vi "Example of fetch current git version code.vi"() -> ()   [LabVIEW 2016]
panel:
  out "Fetch error?":bool
  out "error out":errorcluster
  out "Version:":string
  # "Run the VI to get version code from the most recent tag with\ngit describe command in this containing folder"
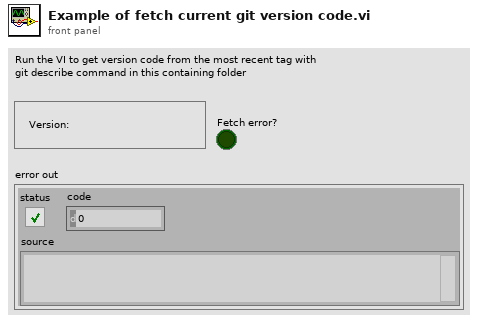
[diagram p1: front panel]
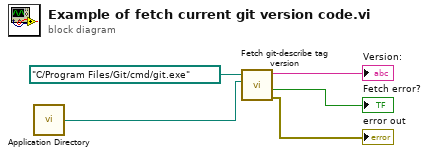
[diagram p0: block diagram]
diagram:
  n1 = call <vilib>:"Application Directory.vi"() -> ("Application Directory"=w1:path)
  n2 = call "Fetch git-describe tag version.vi"("git repo path"=w1, "git.exe path"=path "C:/Program Files/Git/cmd/git.exe") -> ("error out"=→"error out":errorcluster, "Fetch error?"=→"Fetch error?":bool, "Version string"=→"Version:":string)  [unwired: 6 in, 1 out]
